vi "ZCAN_InitCAN(PCIeFD).vi"(0 "device_hande":u32, 1 "filter":u8, 2 "acc_code":u32, 3 "acc_mask":u32, 5 "can_index":u32, 7 "baudrate":u32, 9 "mode":u8, 11 "error in (no error)":errorcluster caption="错误输入（无错误）", 12 "baud_rate_custom？":bool, 13 "RateCustom":string) -> (8 "can_index_handle":u32, 15 "error out":errorcluster caption="错误输出")   [LabVIEW 2018]
uses:
  bin/zlgcan_wrap.dll
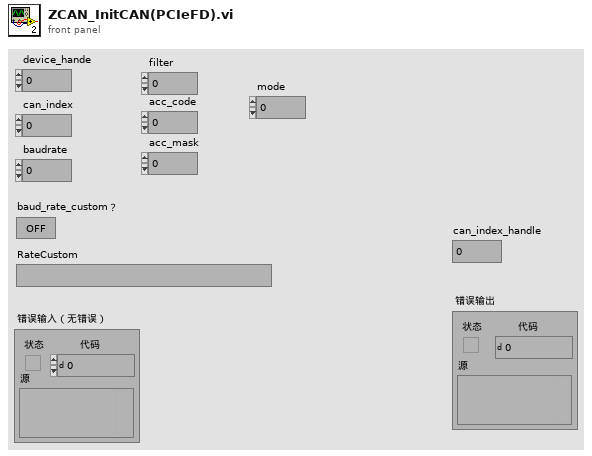
[diagram p1: front panel]
types:
  T1 = cluster{"can_type":u32, "acc_code":u32, "acc_mask":u32, "can_type":u32, "can_type":u32, "can_type":u32, "filter":u8, "mode":u8, "pad":u16, "reserved":u32}
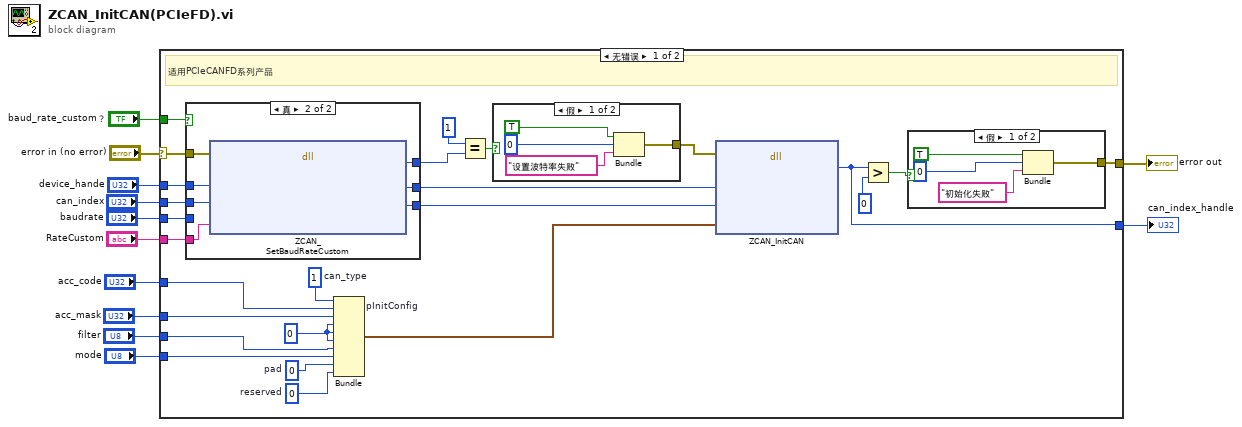
[diagram p0: block diagram]
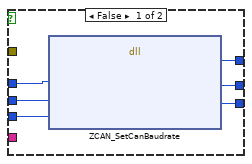
[diagram p4: hidden frame]
diagram:
  n1 = case shown="无错误" "error in (no error)" {
    selector: "error in (no error)" -> [w31 w59]
    tunnel: [w30 w59] -> w11
    tunnel: "baud_rate_custom？" -> [w37 _]
    tunnel: "device_hande" -> [w36 _]
    tunnel: "can_index" -> [w35 _]
    tunnel: "baudrate" -> [w34 _]
    tunnel: "RateCustom" -> [w33 _]
    tunnel: "mode" -> [w32 _]
    tunnel: [w29 _] -> w4
    tunnel: "acc_code" -> [w28 _]
    tunnel: "acc_mask" -> [w27 _]
    tunnel: "filter" -> [w26 _]
    frame No Error {
      w13 = u32 0  # reserved
      w14 = u16 0  # pad
      w15 = u32 0 ("can_type")
      w17 = u32 1  # can_type
      # "适用PCIeCANFD系列产品"
      n2 = case shown="真" w37 {
        tunnel: [w50 w58] -> w25
        tunnel: [w49 w57] -> w24
        tunnel: [w51 w56] -> w22
        tunnel: w36 -> [w48 w54]
        tunnel: w35 -> [w47 w53]
        tunnel: w34 -> [w46 _]
        tunnel: w33 -> [_ w55]
        tunnel: w31 -> [_ w52]
        frame False {
          n3 = dll-call lib="D:/USBCANFD DEMO/zlgcan_wrap_20191223/bin/zlgcan_wrap.dll" fn="ZCAN_SetCanBaudrate"("hDev"=w48, "can_index"=w47, "baudrate"=w46) -> ("return"=w51:u32, "hDev"=w50:u32, "can_index"=w49:u32)  [unwired: 4 in, 2 out]
        }
        frame True {
          n4 = dll-call lib="D:/USBCANFD DEMO/zlgcan_wrap_20191223/bin/zlgcan_wrap.dll" fn="ZCAN_SetBaudRateCustom"(error in=w52, "device_handle"=w54, "can_index"=w53, "RateCustom"=w55) -> ("return"=w56:u32, "device_handle"=w58:u32, "can_index"=w57:u32)  [unwired: 3 in, 2 out]
        }
      }
      n5 = Bundle "pInitConfig"("can_type"=w17, "acc_code"=w28, "acc_mask"=w27, "can_type"=w15, "can_type"=w15, "can_type"=w15, "filter"=w26, "mode"=w32, "pad"=w14, "reserved"=w13) -> (w16:T1)  [unwired: 1 in]
      n6 = Equal?(x=1, y=w22) -> (x = y?=w21:bool)
      n7 = case shown="假" w21 {
        tunnel: [w42 _] -> w20
        frame False {
          n8 = Bundle("status"=TRUE, "code"=0, "消息"="设置波特率失败") -> (w42:cluster{"status":bool, "code":i32, "消息":string})  [unwired: 1 in]
        }
        frame True {
        }
      }
      n9 = dll-call lib="D:/USBCANFD DEMO/zlgcan_wrap_20191223/bin/zlgcan_wrap.dll" fn="ZCAN_InitCAN"(error in=w20, "device_handle"=w25, "can_index"=w24, "pInitConfig"=w16) -> ("can_handle"=w29:u32)  [unwired: 5 in, 2 out]
      n10 = Greater?(x=w29, y=0) -> (0:w18:bool)
      n11 = case shown="假" w18 {
        tunnel: [w38 _] -> w30
        frame False {
          n12 = Bundle("status"=TRUE, "code"=0, "消息"="初始化失败") -> (w38:cluster{"status":bool, "code":i32, "消息":string})  [unwired: 1 in]
        }
        frame True {
        }
      }
    }
    frame Error {
    }
  }
  "error out" <- w11
  "can_index_handle" <- w4
